vi "出栈.vi"(8 "error in (no error)":errorcluster caption="错误输入（无错误）", 11 "堆栈(DBL) 输入":refnum<class "堆栈(CTRL-REF).lvclass"> caption="DNL_LabVIEW Object in") -> (0 "error out":errorcluster caption="错误输出", 1 "堆栈空":bool, 2 "元素":refnum<vi>, 3 "堆栈(DBL) 输出":refnum<class "堆栈(CTRL-REF).lvclass"> caption="DNL_LabVIEW Object out")   [LabVIEW 2011, in "堆栈(CTRL-REF).lvclass"]
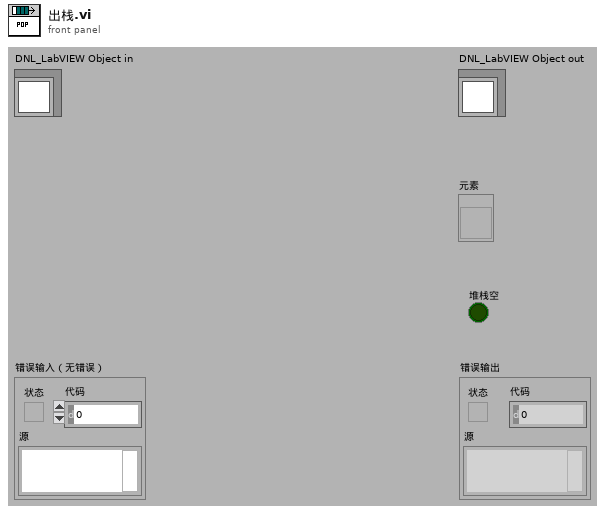
[diagram p1: front panel]
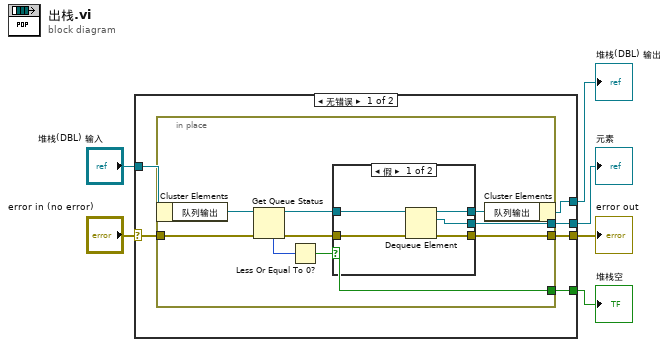
[diagram p0: block diagram]
diagram:
  n1 = case shown="无错误" "error in (no error)" {
    selector: "error in (no error)" -> [w9 w30]
    tunnel: [w8 w30] -> w5
    tunnel: [w11 w29] -> w3
    tunnel: "堆栈(DBL) 输入" -> [w12 w29]
    tunnel: [w10 _] -> w2
    tunnel: [w7 _] -> w1
    frame No Error {
      n2 = in-place {
        in-place-border: [w19] -> w10
        in-place-border: w9 -> [w17]
        in-place-border: [w16] -> w8
        in-place-border: [w13] -> w7
        n3 = in-place-cluster #1(w12) -> ("队列输出"=w21:refnum<queue>)
        n4 = Get Queue Status(queue=w21, error in (no error)=w17) -> (queue out=w15:refnum<queue>, error out=w18:errorcluster, # elements in queue=w20:i32)  [unwired: 1 in, 5 out]
        n5 = Less Or Equal To 0?(x=w20) -> (x <= 0?=w19:bool)
        n6 = case shown="假" w19 {
          tunnel: w18 -> [w24 w28]
          tunnel: [w23 w28] -> w16
          tunnel: w15 -> [w26 w27]
          tunnel: [w25 w27] -> w14
          tunnel: [w22 _] -> w13
          frame False {
            n7 = Dequeue Element(queue=w26, error in (no error)=w24) -> (queue out=w25:refnum<queue>, element=w22:refnum<vi>, error out=w23:errorcluster)  [unwired: 1 in, 1 out]
          }
          frame True {
          }
        }
        n8 = in-place-cluster #1("队列输出"=w14) -> (w11:refnum<class "堆栈(CTRL-REF).lvclass">)
      }
    }
    frame Error {
    }
  }
  "error out" <- w5
  "堆栈(DBL) 输出" <- w3
  "元素" <- w1
  "堆栈空" <- w2
